vi "Motion@Config__Parameter.vi"(1 "ParamterIn":string) -> (0 "ParamterOut":string)   [LabVIEW 2020]
panel:
  in  "Axis":string(combo)="X"
  in  "Value":string(combo)
  in  "Parameter":string(combo)="Scale"
  in  "MotorName":string(combo)
  in  "Confirm":bool
  # "Motor@Config $Motor,$Axis,$Parameter,$Value"
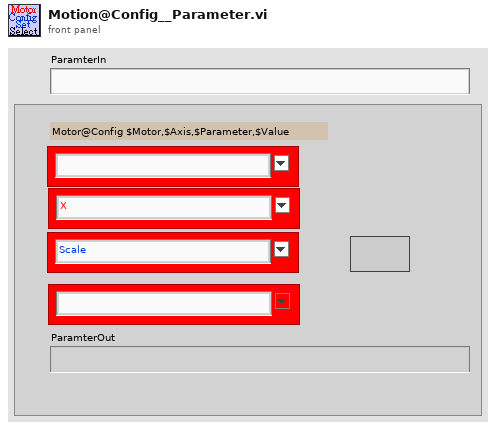
[diagram p1: front panel]
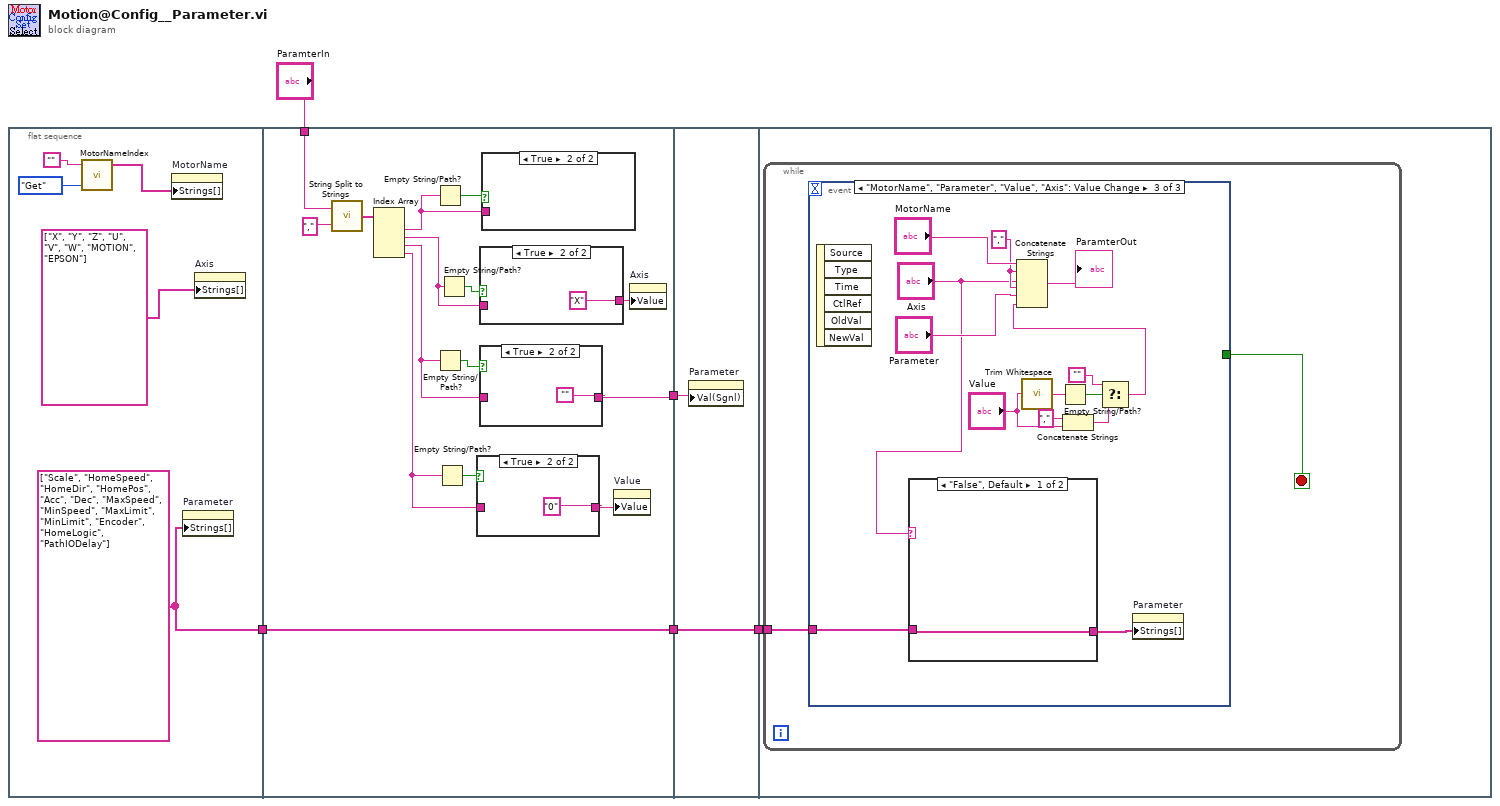
[diagram p0: block diagram]
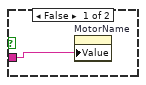
[diagram p5: hidden frame]
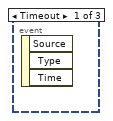
[diagram p6: hidden frame]
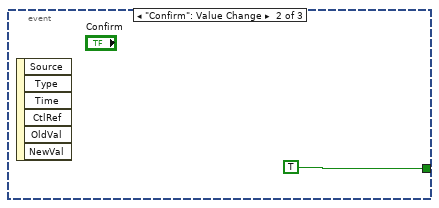
[diagram p7: hidden frame]
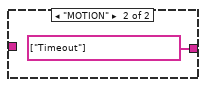
[diagram p8: hidden frame]
diagram:
  n1 = flat-sequence {
    tunnel: [w6] -> w1
    tunnel: "ParamterIn" -> [w23]
    tunnel: [w17] -> w4
    tunnel: [w12] -> w2
    tunnel: w1 -> [w12]
    tunnel: w4 -> [w34]
    tunnel: [w33] -> w3
    tunnel: w2 -> [w33]
    tunnel: w3 -> [w35]
    frame #0 {
      w6 = string[] ["Scale", "HomeSpeed", "HomeDir", "HomePos", "Acc", "Dec", "MaxSpeed", "MinSpeed", "MaxLimit", "MinLimit", "Encoder", "HomeLogic", "PathIODelay"]
      n2 = call "MotorNameIndex.vi"("OP"=enum16{"Get", "Update", "Init"}."Get", "MotorName"="") -> ("MotorList"=w8:string[])  [unwired: 1 in, 2 out]
      n3 = property on="MotorName" class="CmbBox"("Strings[]"=w8) -> ()  [unwired: 2 in, 2 out]
      n4 = property on="Parameter" class="CmbBox"("Strings[]"=w6) -> ()  [unwired: 2 in, 2 out]
      n5 = property on="Axis" class="CmbBox"("Strings[]"=string[] ["X", "Y", "Z", "U", "V", "W", "MOTION", "EPSON"] ("Strings []")) -> ()  [unwired: 2 in, 2 out]
    }
    frame #1 {
      n6 = call "String Split to Strings.vi"("search string/char (-)"=",", "String"=w23) -> ("Array"=w25:string[])
      n7 = Index Array(array=w25) -> (element #1=w21:string, element #2=w13:string, element #3=w15:string, element #4=w16:string)  [unwired: 4 in]
      n8 = Empty String/Path?(string/path=w21) -> (empty?=w22:bool)
      n9 = Empty String/Path?(string/path=w15) -> (empty?=w20:bool)
      n10 = Empty String/Path?(string/path=w16) -> (empty?=w19:bool)
      n11 = Empty String/Path?(string/path=w13) -> (empty?=w14:bool)
      n12 = case shown="True" w19 {
        tunnel: [w28 "0"] -> w18
        tunnel: w16 -> [w28 _]
        frame False {
        }
        frame True {
        }
      }
      n13 = case shown="True" w14 {
        tunnel: w13 -> [w26 _]
        tunnel: [w26 "X"] -> w11
        frame False {
        }
        frame True {
        }
      }
      n14 = case shown="True" w20 {
        tunnel: [w30 ""] -> w17
        tunnel: w15 -> [w30 _]
        frame False {
        }
        frame True {
        }
      }
      n15 = case shown="True" w22 {
        tunnel: w21 -> [w32 _]
        frame False {
          n16 = property on="MotorName" class="CmbBox"("Value"=w32) -> ()  [unwired: 2 in, 2 out]
        }
        frame True {
        }
      }
      n17 = property on="Value" class="CmbBox"("Value"=w18) -> ()  [unwired: 2 in, 2 out]
      n18 = property on="Axis" class="CmbBox"("Value"=w11) -> ()  [unwired: 2 in, 2 out]
    }
    frame #2 {
      n19 = property on="Parameter" class="CmbBox"("Val(Sgnl)"=w34) -> ()  [unwired: 2 in, 2 out]
    }
    frame #3 {
      n20 = while {
        tunnel: w35 -> [w36]
        stop <- w37 stop-if-true
        n21 = event shown="[2] \"MotorName\", \"Parameter\", \"Value\", \"Axis\": Value Change" {
          selector: _ -> [_ _ _]
          dyn-events: _ -> [_ _ _]
          timeout: _ -> [_ _ _]
          tunnel: [_ TRUE _] -> w37
          tunnel: w36 -> [_ _ w40]
          event Timeout {
            n22 = event-data() -> ()  [unwired: 1 in, 3 out]
          }
          event "Confirm": Value Change {
            n23 = event-data() -> ()  [unwired: 1 in, 6 out]
          }
          event "MotorName", "Parameter", "Value", "Axis": Value Change {
            w44 = "," ("string")
            n24 = event-data() -> ()  [unwired: 1 in, 6 out]
            n25 = case shown="\"False\", Default" "Axis" {
              tunnel: w40 -> [w53 _]
              tunnel: [w53 string[] ["Timeout"]] -> w39
              frame "False", Default {
              }
              frame "MOTION" {
              }
            }
            n26 = call <vilib>:"Trim Whitespace.vi"("string"="Value") -> ("trimmed string"=w46:string)  [unwired: 1 in]
            n27 = Empty String/Path?(string/path=w46) -> (empty?=w47:bool)
            n28 = Concatenate Strings("," ("string"), "Value") -> (w49:string)
            n29 = Select(t="", s=w47, f=w49) -> (s? t:f=w43:string)
            n30 = Concatenate Strings("MotorName", w44, "Axis", w44, "Parameter", w43) -> (→"ParamterOut":string)
            n31 = property on="Parameter" class="CmbBox"("Strings[]"=w39) -> ()  [unwired: 2 in, 2 out]
          }
        }
      }
    }
  }
